vi "Add Class Documentation.vi"   [LabVIEW 2015]
doc: "<b> </b> <b> </b>\n©2016 Q Software Innovations, LLC (QSI)\nwritten by Quentin Alldredge\nproduced in LabVIEW 2015"
uses:
  Project Manipulation Scripts/Project Manipulation Scripts.lvlib
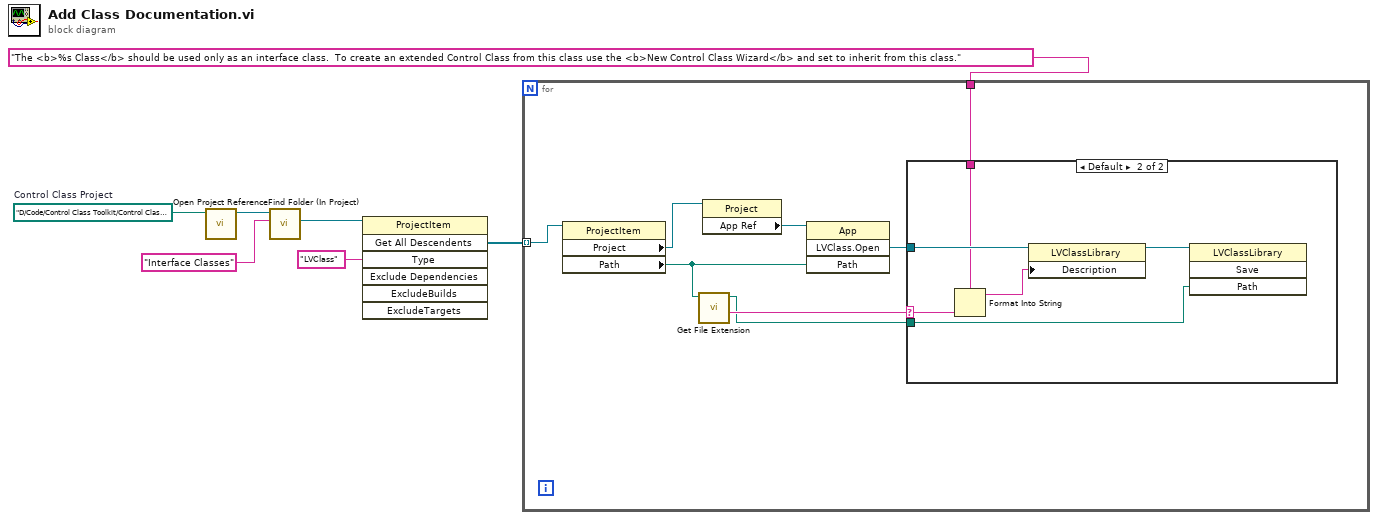
[diagram p0: block diagram]
diagram:
  w7 = path "D:/Code/Control Class Toolkit/Control Class Toolkit.lvproj"  # Control Class Project
  n1 = call "Open Project Reference.vi"("Project Path"=w7) -> ("Project out"=w6:refnum<vi>)  [unwired: 10 in]
  n2 = call "Find Folder (In Project).vi"("Folder Name"="Interface Classes", "Project in"=w6) -> ("Folder Refnum"=w4:refnum<vi>)  [unwired: 7 in, 2 out]
  n3 = invoke class="ProjectItem" method="Get All Descendents"(reference=w4, "Type"="LVClass") -> ("All Descendents"=w2:refnum<vi>[])  [unwired: 5 in, 6 out]
  n4 = for {
    tunnel: w2 -> [w15] mode=indexing
    tunnel: "The <b>%s Class</b> should be used only as an interface class.  To create an extended Control Class from this class use the <b>New Control Class Wizard</b> and set to inherit from this class." ("Type") -> [w10]
    n5 = property class="ProjectItem"(reference=w15) -> ("Project"=w14:refnum<vi>, "Path"=w11:path)  [unwired: 1 in, 2 out]
    n6 = call <vilib>:"Get File Extension.vi"("file"=w11) -> ("filename without extension"=w9:string, "dup file"=w8:path)  [unwired: 6 in, 3 out]
    n7 = property class="Project"(reference=w14) -> ("App Ref"=w13:refnum<vi>)  [unwired: 1 in, 2 out]
    n8 = invoke class="App" method="LVClass.Open"(reference=w13, "Path"=w11) -> ("LVClass.Open"=w12:refnum<vi>)  [unwired: 2 in, 3 out]
    n9 = case shown="Default" w9 {
      selector: w9 -> [_ w19]
      tunnel: w12 -> [_ w21]
      tunnel: w10 -> [_ w20]
      tunnel: w8 -> [_ w16]
      frame "Control" {
      }
      frame Default {
        n10 = Format Into String(format string=w20, w19) -> (resulting string=w18:string)  [unwired: 2 in, 1 out]
        n11 = property class="LVClassLibrary"(reference=w21, "Description"=w18) -> (reference out=w17:refnum<vi>)  [unwired: 1 in, 1 out]
        n12 = invoke class="LVClassLibrary" method="Save"(reference=w17, "Path"=w16) -> ()  [unwired: 2 in, 4 out]
      }
    }
  }
